vi "Save Version.vi"(6 "Top Level/Always Included VIs":path[](array[path]), 7 "Main Destination Path":path, 9 "Target Name":string, 10 "Build Specification Name":string, 11 "Project Path":path) -> (0 "error out":errorcluster)   [LabVIEW 2020]
uses:
  <vilib>/AppBuilder/AB_API_Simple/Get Build Specification Version (path).vi
  <vilib>/AppBuilder/AB_API_Simple/NI_App_Builder_API.lvlib
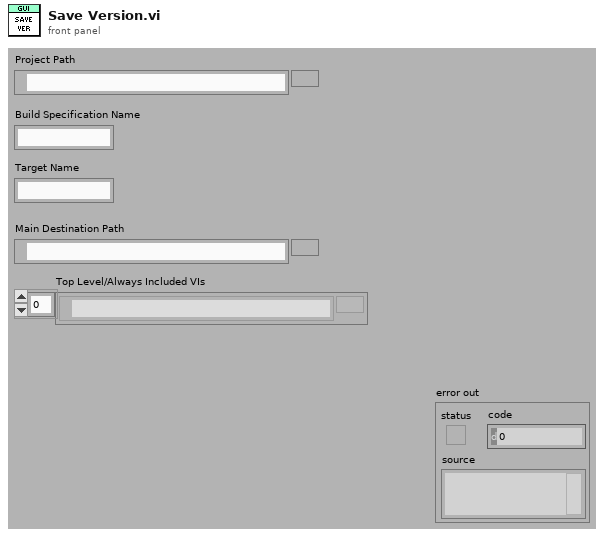
[diagram p1: front panel]
types:
  T1 = enum16{"open", "replace", "create", "open or create", "replace or create", "replace or create with confirmation"}
  T2 = typedef "NI_App_Builder_API.lvlib/Build Specification Version.ctl" = cluster{"Major":u16, "Minor":u16, "Fix":u16, "Build":u16}
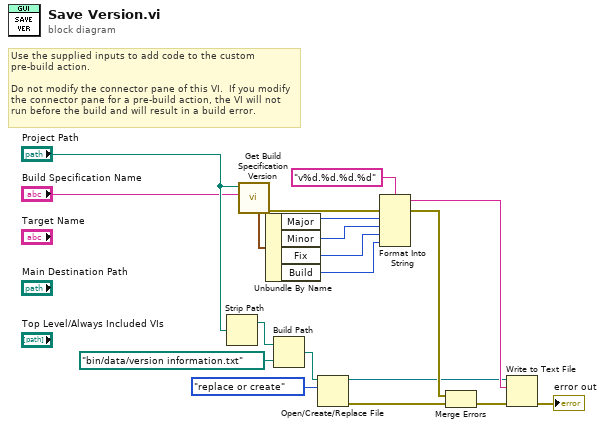
[diagram p0: block diagram]
diagram:
  # "Use the supplied inputs to add code to the custom pre-build action.\n\nDo not modify the connector pane of this VI.  If you modify the connector pane for a pre-build action, the VI will not run before the build and will result in a build error."
  n1 = Strip Path(path="Project Path") -> (stripped path=w4:path)  [unwired: 1 out]
  n2 = call-poly <vilib>:"Get Build Specification Version.vi"("Name of build specification"="Build Specification Name", "Path to project"="Project Path") -> ("error out"=w12:errorcluster, "Build Specification Version"=w18:T2)  [unwired: 8 in]
  n3 = Unbundle By Name(w18) -> ("Major"=w17:u16, "Minor"=w16:u16, "Fix"=w15:u16, "Build"=w14:u16)
  n4 = Build Path(base path=w4, name or relative path=path "bin/data/version information.txt") -> (appended path=w5:path)
  n5 = Open/Create/Replace File(file path (use dialog)=w5, operation (0:open)=T1."replace or create") -> (refnum out=w7:refnum<file>, error out=w6:errorcluster)  [unwired: 4 in, 1 out]
  n6 = Format Into String(format string="v%d.%d.%d.%d", error in=w12, w17, w16, w15, w14) -> (resulting string=w11:string, error out=w9:errorcluster)  [unwired: 1 in]
  n7 = Merge Errors(w9, w6) -> (w10:errorcluster)
  n8 = Write to Text File(file (use dialog)=w7, text=w11, error in=w10) -> (error out=→"error out":errorcluster)  [unwired: 1 in, 2 out]
